vi "HCCTest.vi"   [LabVIEW 2014]
uses:
  c_MicroZedInstr_Enum.ctl
  c_ReportMessages.ctl
  g_MicroZed_Interface.vi
  g_ReportControl.vi
types:
  T1 = typedef "c_MicroZedInstr_Enum.ctl" = enum16{"Start Test Procedure", "Print Instructions", "Config HCC Register", "Send Parameters"}
  T2 = typedef "c_ReportMessages.ctl" = string
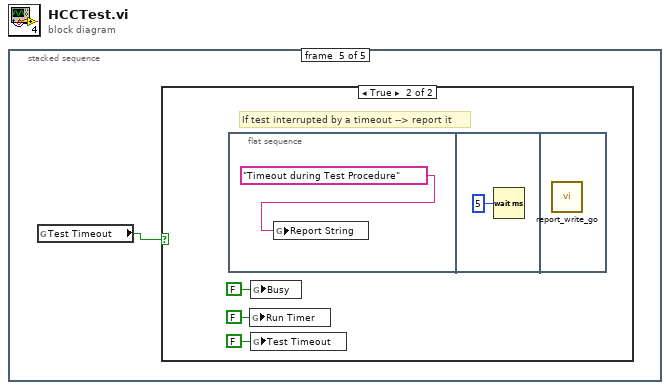
[diagram p0: block diagram]
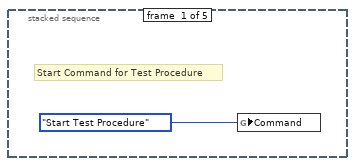
[diagram p2: hidden frame]
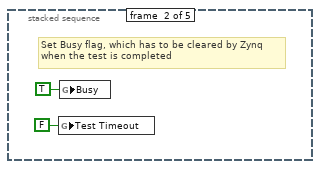
[diagram p3: hidden frame]
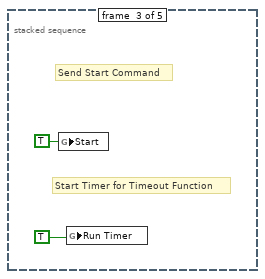
[diagram p4: hidden frame]
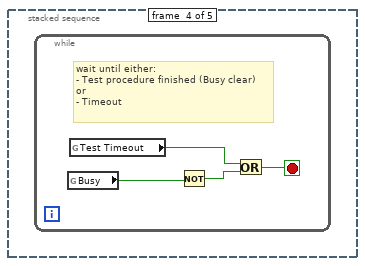
[diagram p5: hidden frame]
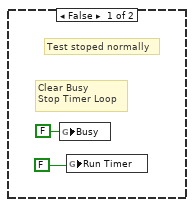
[diagram p6: hidden frame]
diagram:
  n1 = stacked-sequence {
    frame #0 {
      # "Start Command for Test Procedure"
      n2 = global write "g_MicroZed_Interface.vi" "Command"(c_MicroZedInstr_Enum."Start Test Procedure" ("Command")) -> ()
    }
    frame #1 {
      # "Set Busy flag, which has to be cleared by Zynq\nwhen the test is completed"
      n3 = global write "g_MicroZed_Interface.vi" "Test Timeout"(FALSE ("Busy")) -> ()
      n4 = global write "g_MicroZed_Interface.vi" "Busy"(TRUE ("Busy")) -> ()
    }
    frame #2 {
      # "Start Timer for Timeout Function"
      # "Send Start Command"
      n5 = global write "g_MicroZed_Interface.vi" "Start"(TRUE ("Start")) -> ()
      n6 = global write "g_MicroZed_Interface.vi" "Run Timer"(TRUE ("Start")) -> ()
    }
    frame #3 {
      n7 = while {
        stop <- w6 stop-if-true
        # "wait until either:\n- Test procedure finished (Busy clear)\nor\n- Timeout"
        n8 = global read "g_MicroZed_Interface.vi" "Busy"() -> (w8:bool)
        n9 = global read "g_MicroZed_Interface.vi" "Test Timeout"() -> (w7:bool)
        n10 = Not(x=w8) -> (.not. x?=w9:bool)
        n11 = Or(x=w7, y=w9) -> (x .or. y?=w6:bool)
      }
    }
    frame #4 {
      n12 = global read "g_MicroZed_Interface.vi" "Test Timeout"() -> (w10:bool)
      n13 = case shown="True" w10 {
        frame False {
          # "Test stoped normally"
          # "Clear Busy\nStop Timer Loop"
          n14 = global write "g_MicroZed_Interface.vi" "Busy"(FALSE ("Busy")) -> ()
          n15 = global write "g_MicroZed_Interface.vi" "Run Timer"(FALSE ("Start")) -> ()
        }
        frame True {
          # "If test interrupted by a timeout --> report it"
          n16 = flat-sequence {
            frame #0 {
              n17 = global write "g_ReportControl.vi" "Report String"(T2 "Timeout during Test Procedure" ("Combo Box")) -> ()
            }
            frame #1 {
              n18 = Wait (ms)(milliseconds to wait=u32 5) -> ()  [unwired: 1 out]
            }
            frame #2 {
              n19 = call "report_write_go.vi"() -> ()  [unwired: 12 in]
            }
          }
          n20 = global write "g_MicroZed_Interface.vi" "Run Timer"(FALSE ("Start")) -> ()
          n21 = global write "g_MicroZed_Interface.vi" "Busy"(FALSE ("Busy")) -> ()
          n22 = global write "g_MicroZed_Interface.vi" "Test Timeout"(FALSE ("Test Timeout")) -> ()
        }
      }
    }
  }
